vi "Size.vi"(0 "State In":T1, 1 "XRef":refnum<vi>, 3 "Bounds":T13) -> (2 "State Out":T1, 4 "Reply":string[](array[string]))   [LabVIEW 2012]
uses:
  State.ctl
  <vilib>/picture/picture.llb/imagedata.ctl
  <vilib>/XNodeSupport/XNodeTerm3Array.ctl
  <vilib>/XNodeSupport/XNodeTerm3.ctl
  <vilib>/XNodeSupport/XNodeString.ctl
  <vilib>/XNodeSupport/XNodeVariant.ctl
  <vilib>/XNodeSupport/XNodeRect32.ctl
  <vilib>/XNodeSupport/XNodeInt.ctl
  <vilib>/XNodeSupport/XNodeBool.ctl
  <vilib>/XNodeSupport/XNodeTermDirection.ctl
  Subvis/Term Types.ctl
  Subvis/Term Type.ctl
  <vilib>/XNodeSupport/NI_XNodeSupport.lvlib
  ConPane Wrapper.xnode
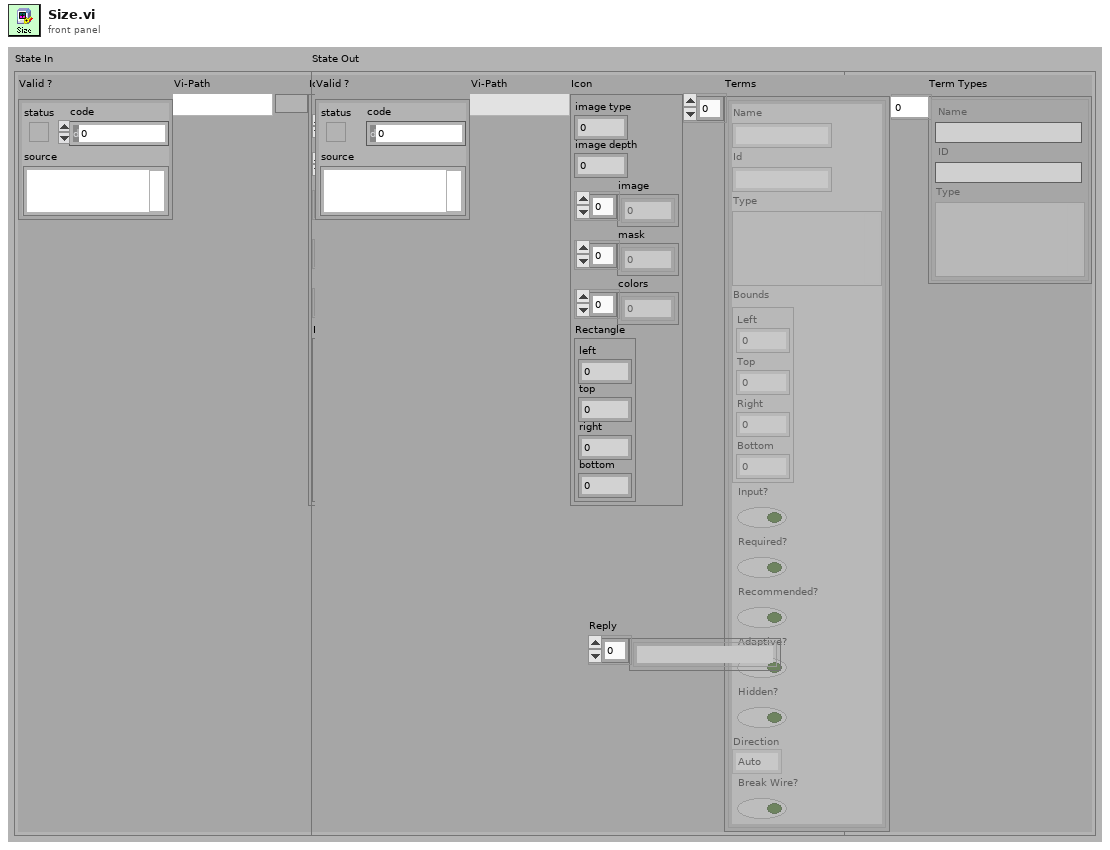
[diagram p1: front panel]
types:
  T1 = typedef "ConPane Wrapper.xnode/State.ctl" = cluster{"Valid ?":errorcluster, "Vi-Path":path, "Icon":T2, "Terms":T3, "Term Types":T11}
  T2 = typedef "imagedata.ctl" = cluster{"image type":i32, "image depth":i32, "image":u8[], "mask":u8[], "colors":u32[], "Rectangle":cluster{"left":i16, "top":i16, "right":i16, "bottom":i16}}
  T3 = typedef "NI_XNodeSupport.lvlib/XNodeTerm3Array.ctl" = T4[]
  T4 = typedef "NI_XNodeSupport.lvlib/XNodeTerm3.ctl" = cluster{"Name":T5, "Id":T5, "Type":T6, "Bounds":T7, "Input?":T9, "Required?":T9, "Recommended?":T9, "Adaptive?":T9, "Hidden?":T9, "Direction":T10, "Break Wire?":T9}
  T5 = typedef "NI_XNodeSupport.lvlib/XNodeString.ctl" = string
  T6 = typedef "NI_XNodeSupport.lvlib/XNodeVariant.ctl" = variant
  T7 = typedef "NI_XNodeSupport.lvlib/XNodeRect32.ctl" = cluster{"Left":T8, "Top":T8, "Right":T8, "Bottom":T8}
  T8 = typedef "NI_XNodeSupport.lvlib/XNodeInt.ctl" = i32
  T9 = typedef "NI_XNodeSupport.lvlib/XNodeBool.ctl" = bool
  T10 = typedef "NI_XNodeSupport.lvlib/XNodeTermDirection.ctl" = enum32{"Auto", "Up", "Down", "Left", "Right", "Center"}
  T11 = typedef "Term Types.ctl" = T12[]
  T12 = typedef "Term Type.ctl" = cluster{"Name":string, "ID":string, "Type":variant}
  T13 = cluster{"Left":T8, "Top":T8, "Right":T8, "Bottom":T8}
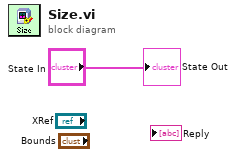
[diagram p0: block diagram]
diagram:
  "State Out" <- "State In"
